vi "DriverStation Set User Code Runningvi.vi"(8 "error in (no error)":errorcluster, 11 "code ready for enable":bool) -> (0 "error out":errorcluster)   [LabVIEW 2026, in "MrcLib.lvlib"]
doc: "Update the DS and FMS with the state of the robot code"
uses:
  MrcLib.lvlib
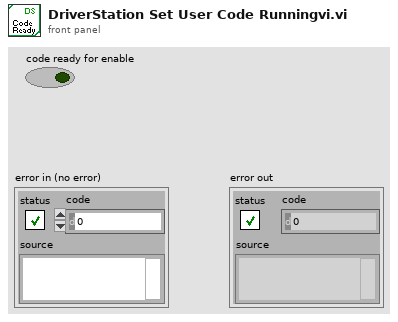
[diagram p1: front panel]
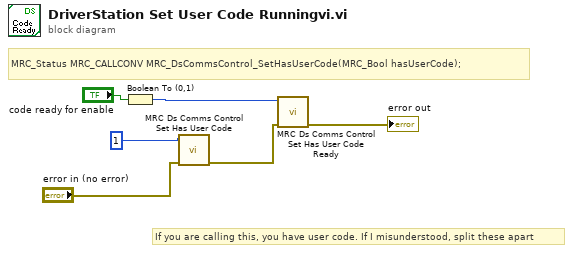
[diagram p0: block diagram]
diagram:
  # "If you are calling this, you have user code. If I misunderstood, split these apart"
  # "MRC_Status MRC_CALLCONV MRC_DsCommsControl_SetHasUserCode(MRC_Bool hasUserCode);"
  n1 = Boolean To (0,1)(Boolean="code ready for enable") -> (0, 1=w2:i16)
  n2 = call "MRC Ds Comms Control Set Has User Code.vi"("error in (no error)"="error in (no error)", "hasUserCode"=u8 1) -> ("error out"=w4:errorcluster)  [unwired: 9 in]
  n3 = call "MRC Ds Comms Control Set Has User Code Ready.vi"("error in (no error)"=w4, "hasUserCodeReady"=w2) -> ("error out"=→"error out":errorcluster)  [unwired: 9 in]
